vi "HaltSkill_v2_Init.vi"(0 "object in":refnum<class "HaltSkill_v2.lvclass">, 5 "error in (no error)":errorcluster) -> (14 "object out":refnum<class "HaltSkill_v2.lvclass">, 19 "error out":errorcluster)   [LabVIEW 2023, in "HaltSkill_v2.lvclass"]
uses:
  HaltSkill_v2.lvclass
  C:/Users/ebert/Documents/codes/SSL/repo/SSL_AI/NewSTP/NewSkills/Skill_v2_class/Skill_v2.lvclass
  HaltSkill_v2.lvclass/HaltSkill_v2.ctl
  Skill_v2_class/Skill_v2.lvclass
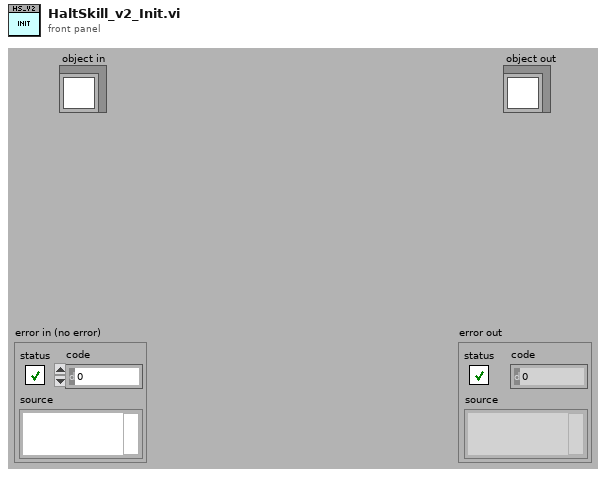
[diagram p1: front panel]
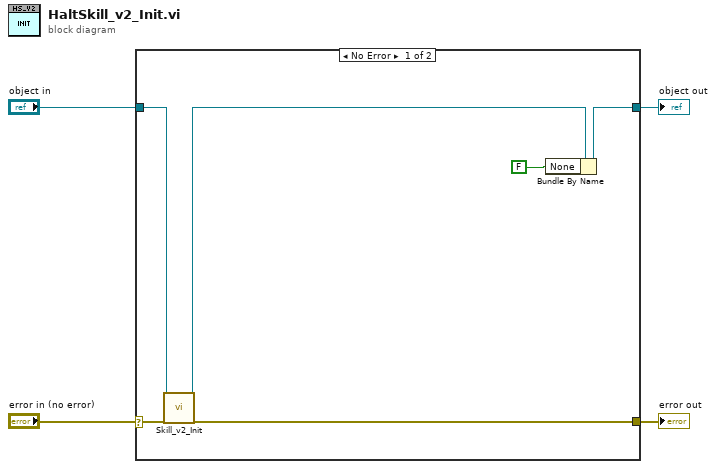
[diagram p0: block diagram]
diagram:
  n1 = case shown="No Error" "error in (no error)" {
    selector: "error in (no error)" -> [w8 w11]
    tunnel: [w10 w12] -> w4
    tunnel: "object in" -> [w6 w12]
    tunnel: [w7 w11] -> w1
    frame No Error {
      n2 = call "Skill_v2_Init.vi"("object in"=w6, "error in (no error)"=w8) -> ("object out"=w5:refnum<class "HaltSkill_v2.lvclass">, "error out"=w7:errorcluster)  [unwired: 16 in]
      n3 = Bundle By Name(cluster=w5, "None"=FALSE) -> (w10:refnum<class "HaltSkill_v2.lvclass">)
    }
    frame Error {
    }
  }
  "object out" <- w4
  "error out" <- w1
